vi "Write Parameter Values.vi"(8 "error in (no error)":errorcluster, 10 "Parameter Values":string[](array[string]), 11 "WriteCommand in":refnum<class "WriteCommand.lvclass">) -> (0 "error out":errorcluster, 3 "WriteCommand out":refnum<class "WriteCommand.lvclass">)   [LabVIEW 2023, in "HAF.lvlib" / "WriteCommand.lvclass"]
doc: "Adds a collection of raw execution results into the Parameters in matched sequence order."
uses:
  WriteCommand.lvclass
  WriteCommand.lvclass/WriteCommand.ctl
  Parameter/Parameter.lvclass
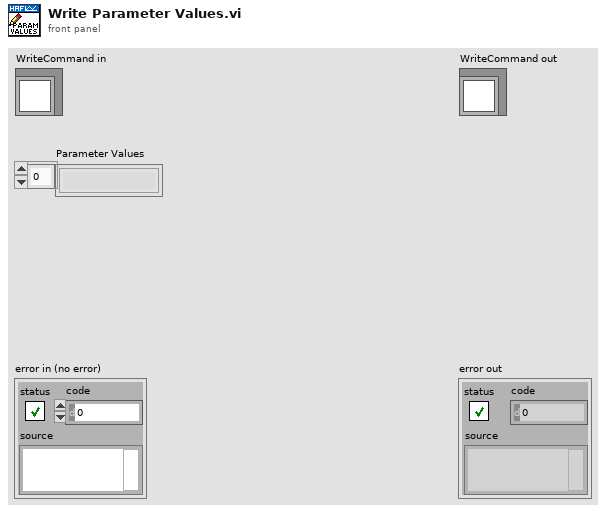
[diagram p1: front panel]
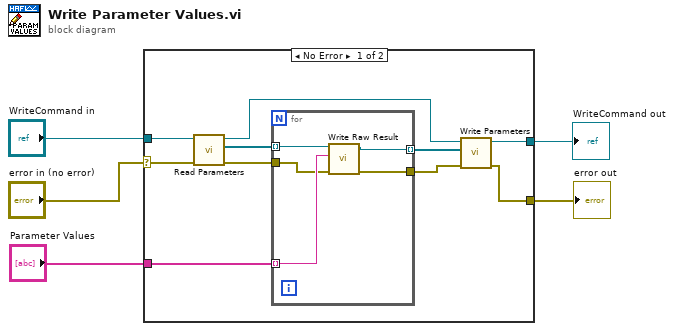
[diagram p0: block diagram]
diagram:
  n1 = case shown="No Error" "error in (no error)" {
    selector: "error in (no error)" -> [w14 w22]
    tunnel: [w6 w22] -> w4
    tunnel: [w7 w21] -> w2
    tunnel: "WriteCommand in" -> [w15 w21]
    tunnel: "Parameter Values" -> [w11 _]
    frame No Error {
      n2 = call-dynamic "Read Parameters.vi"("error in (no error)"=w14, "WriteCommand in"=w15) -> ("error out"=w12:errorcluster, "Parameters"=w13:refnum<class "Parameter.lvclass">[], "WriteCommand out"=w8:refnum<class "WriteCommand.lvclass">)  [unwired: 7 in]
      n3 = for {
        tunnel: w13 -> [w20] mode=indexing
        tunnel: w12 -> [w18]
        tunnel: w11 -> [w19] mode=indexing
        tunnel: [w17] -> w10 mode=indexing
        tunnel: [w16] -> w9
        n4 = call-dynamic "Write Raw Result.vi"("error in (no error)"=w18, "Raw Result"=w19, "Parameter in"=w20) -> ("error out"=w16:errorcluster, "Parameter out"=w17:refnum<class "Parameter.lvclass">)  [unwired: 7 in]
      }
      n5 = call-dynamic "Write Parameters.vi"("error in (no error)"=w9, "Parameters"=w10, "WriteCommand in"=w8) -> ("error out"=w6:errorcluster, "WriteCommand out"=w7:refnum<class "WriteCommand.lvclass">)  [unwired: 7 in]
    }
    frame Error {
    }
  }
  "error out" <- w4
  "WriteCommand out" <- w2
